vi "WT1800 Build Function Name List.vi"(9 "Functions To Retreive":string[](array[string]), 11 "Number of Channels":i32) -> (3 "Array out":string[](array[string]))   [LabVIEW 2021]
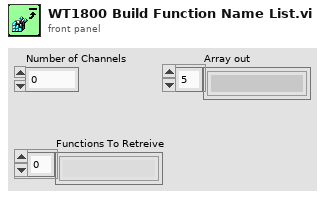
[diagram p1: front panel]
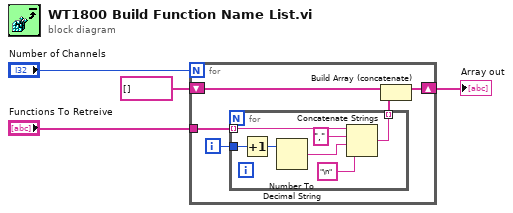
[diagram p0: block diagram]
diagram:
  n1 = for {
    N: "Number of Channels" -> [_]
    shift-right: [w6] -> w3
    shift-left: string[] [] -> [w5]
    tunnel: "Functions To Retreive" -> [w7]
    i -> [w9]
    n2 = for {
      tunnel: w7 -> [w14] mode=indexing
      tunnel: w9 -> [w13]
      tunnel: [w12] -> w8 mode=indexing
      n3 = Increment(x=w13) -> (x+1=w16:i32)
      n4 = Number To Decimal String(number=w16) -> (decimal integer string=w15:string)  [unwired: 1 in]
      n5 = Concatenate Strings(w14, "," ("string"), w15, "\n" ("string")) -> (w12:string)
    }
    n6 = Build Array (concatenate)(w5, w8) -> (w6:string[])
  }
  "Array out" <- w3
